vi "FP - Refresh Datalist_SubVIs-某型振动实验台测试系统.vi"(7 "chn1":refnum<vi>, 8 "error in":errorcluster, 11 "Accele":T1[](array[typedef])) -> (0 "error out":errorcluster, 2 "unit":string[](array[string]))   [LabVIEW 2011]
doc: "Use this template to build a VI to use as a subVI."
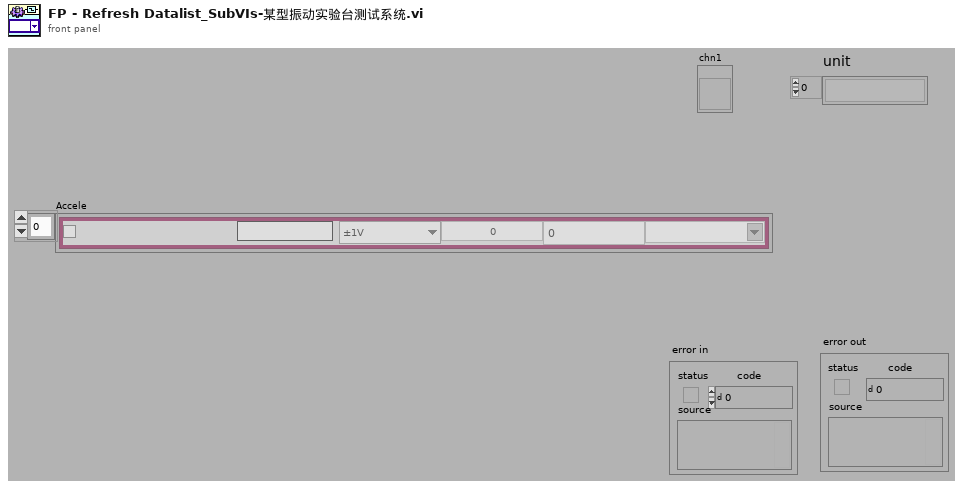
[diagram p1: front panel]
types:
  T1 = typedef "Acceleration Channel Config_Ctrls-某型振动实验台测试系统.ctl" = cluster{"Enable":bool, "Name":string, "range":enum16{"±1V", "±5V"}, "SensValue":dbl, "PhysicalName":string, "off":dbl, "Sensunits":string}
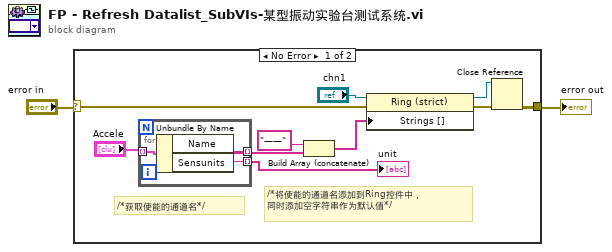
[diagram p0: block diagram]
diagram:
  n1 = case shown="No Error" "error in" {
    selector: "error in" -> [w4 w16]
    tunnel: [w7 w16] -> w1
    frame No Error {
      # "/*将使能的通道名添加到Ring控件中，\n同时添加空字符串作为默认值*/"
      # "/*获取使能的通道名*/"
      n2 = for {
        tunnel: "Accele" -> [w15] mode=indexing
        tunnel: [w14] -> w6 mode=indexing
        tunnel: [w13] -> w3 mode=indexing
        n3 = Unbundle By Name(w15) -> ("Name"=w14:string, "Sensunits"=w13:string)
      }
      "unit" <- w3
      n4 = Build Array (concatenate)("——", w6) -> (w11:string[])
      n5 = property class="Ring (strict)"(reference="chn1", error in=w4, "Strings []"=w11) -> (reference out=w10:refnum<vi>, error out=w8:errorcluster)
      n6 = Close Reference(reference=w10, error in (no error)=w8) -> (error out=w7:errorcluster)
    }
    frame Error {
    }
  }
  "error out" <- w1
